vi "ZDataVIS_Select_Intensity.vi"(5 "B":T2(ring), 7 "A":T2(ring), 8 "error in (no error)":errorcluster, 9 "Slow Index (Row)":dbl, 10 "Slowest Index (Page)":i32, 11 "Big Ol Array IN":T1(array[cluster])) -> (0 "error out":errorcluster, 3 "Intensity Info OUT":cluster{dbl[], dbl[]}[](array[cluster]))   [LabVIEW 2016]
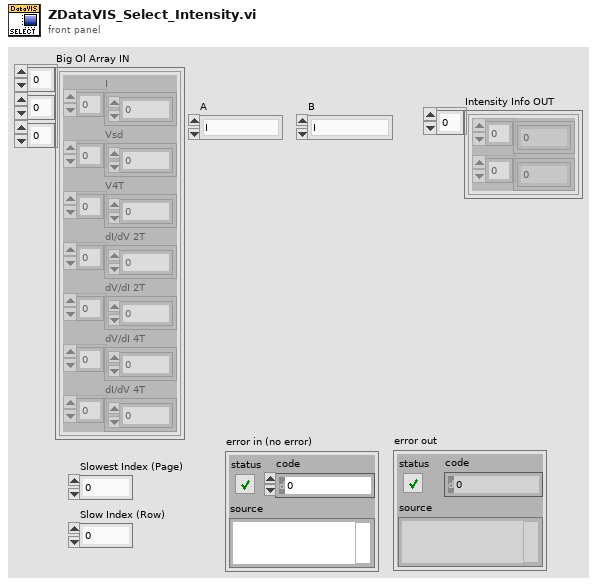
[diagram p1: front panel]
types:
  T1 = cluster{"I":dbl[], "Vsd":dbl[], "V4T":dbl[], "dI/dV 2T":dbl[], "dV/dI 2T":dbl[], "dV/dI 4T":dbl[], "dI/dV 4T":dbl[]}[][][]
  T2 = enum16{"I", "Vsd", "V4T", "dI/dV 2T", "dV/dI 2T", "dV/dI 4T", "dI/dV 4T"}
  T3 = cluster{"I":dbl[], "Vsd":dbl[], "V4T":dbl[], "dI/dV 2T":dbl[], "dV/dI 2T":dbl[], "dV/dI 4T":dbl[], "dI/dV 4T":dbl[]}[]
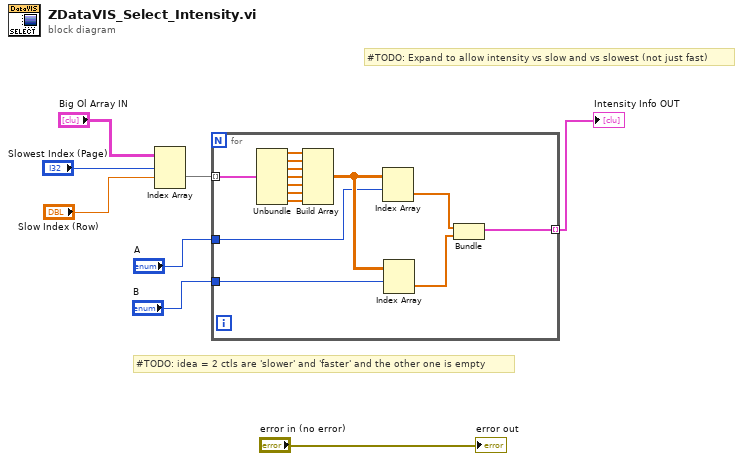
[diagram p0: block diagram]
diagram:
  # "#TODO: idea = 2 ctls are 'slower' and 'faster' and the other one is empty"
  # "#TODO: Expand to allow intensity vs slow and vs slowest (not just fast)"
  n1 = Index Array(array="Big Ol Array IN", index (dim 0)="Slowest Index (Page)", index (dim 1)="Slow Index (Row)") -> (element=w4:T3)  [unwired: 1 in]
  n2 = for {
    tunnel: w4 -> [w15] mode=indexing
    tunnel: [w11] -> w5 mode=indexing
    tunnel: "A" -> [w10]
    tunnel: "B" -> [w9]
    n3 = Unbundle(w15) -> ("I"=w22:dbl[], "Vsd"=w21:dbl[], "V4T"=w20:dbl[], "dI/dV 2T"=w19:dbl[], "dV/dI 2T"=w18:dbl[], "dV/dI 4T"=w17:dbl[], "dI/dV 4T"=w16:dbl[])
    n4 = Build Array(w22, w21, w20, w19, w18, w17, w16) -> (w14:dbl[][])
    n5 = Index Array(array=w14, index (row)=w10) -> (element=w12:dbl[])  [unwired: 1 in]
    n6 = Index Array(array=w14, index (row)=w9) -> (element=w13:dbl[])  [unwired: 1 in]
    n7 = Bundle(w12, w13) -> (w11:cluster{dbl[], dbl[]})  [unwired: 1 in]
  }
  "Intensity Info OUT" <- w5
  "error out" <- "error in (no error)"
